vi "mainMultiColorWorm_2.vi"() -> ()   [LabVIEW 2017]
uses:
  globalUtilities.vi
  getComputerName.vi
  globalDevices.vi
panel:
  in  "piezo":bool
  in  "etl0_0 (piezo_0)":dbl
  out "curr exp time":dbl
  in  "abort":bool
  out "current image 3":u16[][](graph)
  out "current image 2":u16[][](graph)
  out "current image 1":u16[][](graph)
  out "current image 0":u16[][](graph)
  out "current channel":string
  out "current plane":i32
  in  "Strain name":string
  out "folder name":string
  in  "number of Z planes":i32=25
  in  "height of volume (um)":dbl=30.0
  in  "molecules":T1(array[cluster])=[{"molecule"="BFP", "exposureTimeMultiplier"=1.0}, {"molecule"="CyOFP", "exposureTimeMultiplier"=6.0}, {"molecule"="mCherry", "exposureTimeMultiplier"=4.0}, {"molecule"="mNeptune", "exposureTimeMultiplier"=5.0}]
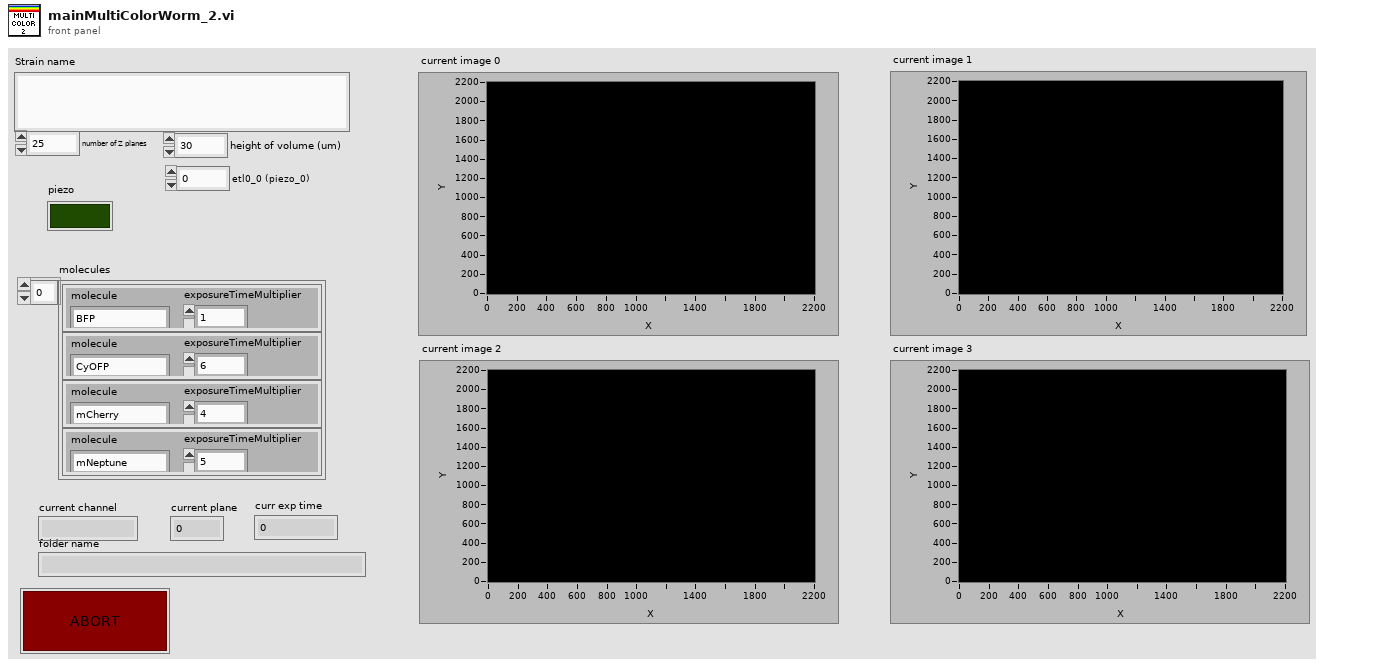
[diagram p1: front panel]
types:
  T1 = cluster{"molecule":string, "exposureTimeMultiplier":dbl}[]
  T2 = cluster{"height":i32, "width":i32, "datatype":i32}
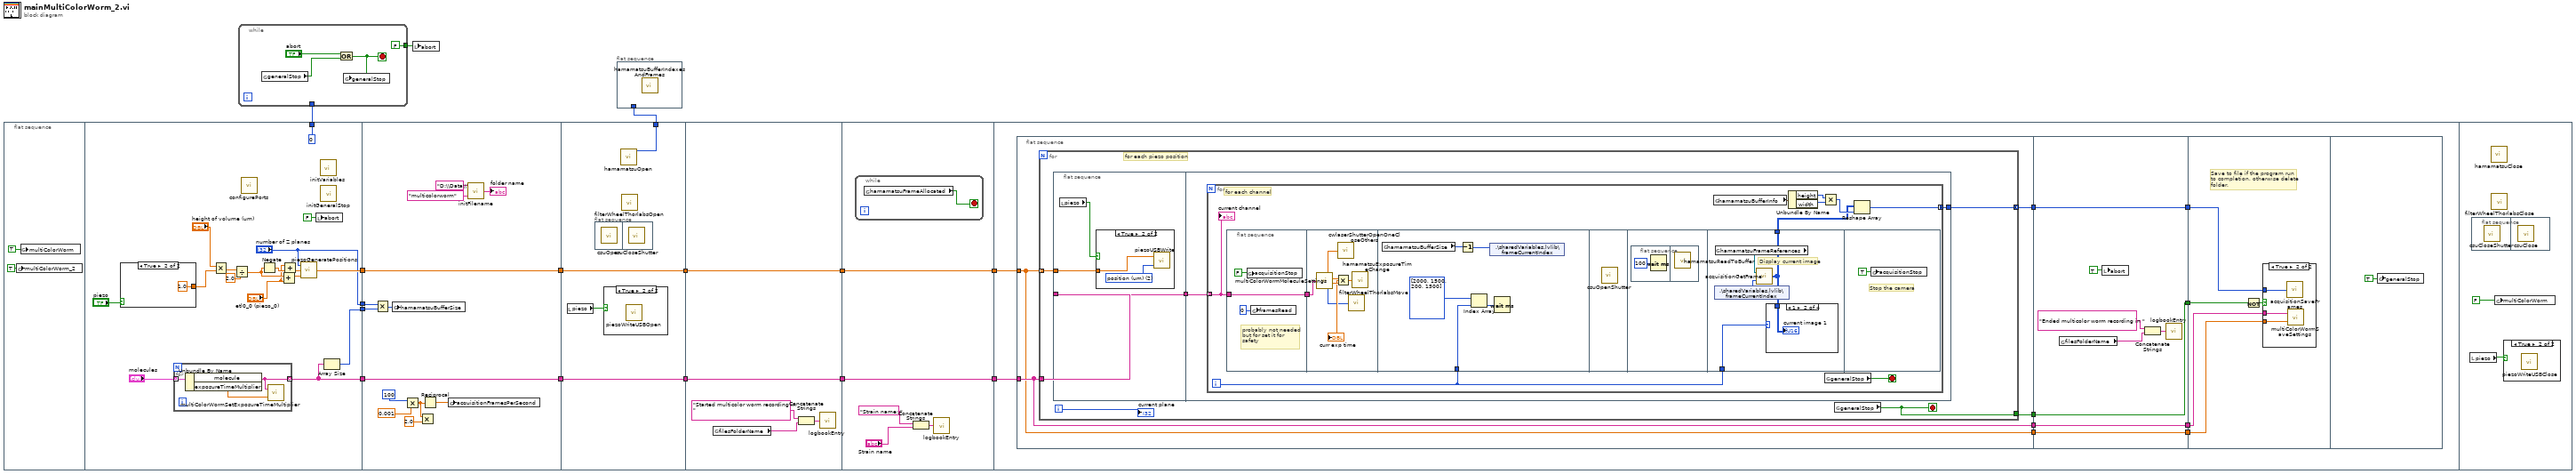
[diagram p0: block diagram]
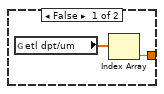
[diagram p2: hidden frame]
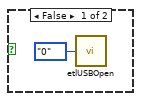
[diagram p3: hidden frame]
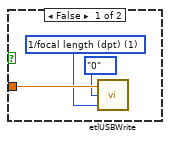
[diagram p4: hidden frame]
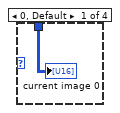
[diagram p5: hidden frame]
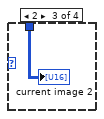
[diagram p6: hidden frame]
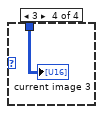
[diagram p7: hidden frame]
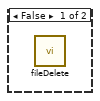
[diagram p8: hidden frame]
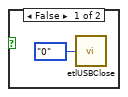
[diagram p9: hidden frame]
diagram:
  n1 = flat-sequence {
    tunnel: [w26] -> w15
    tunnel: [w34] -> w14
    tunnel: ["number of Z planes"] -> w13
    tunnel: [w33] -> w12
    tunnel: [0] -> w2
    tunnel: [w51] -> w11
    tunnel: w15 -> [w51]
    tunnel: [w50] -> w10
    tunnel: w14 -> [w50]
    tunnel: w13 -> [w48]
    tunnel: w12 -> [w47]
    tunnel: [w55] -> w9
    tunnel: [w56] -> w8
    tunnel: [w57] -> w3
    tunnel: w11 -> [w56]
    tunnel: w10 -> [w55]
    tunnel: w9 -> [w63]
    tunnel: [w63] -> w7
    tunnel: w8 -> [w62]
    tunnel: [w62] -> w6
    tunnel: w7 -> [w68]
    tunnel: [w68] -> w5
    tunnel: w6 -> [w67]
    tunnel: [w67] -> w4
    tunnel: w5 -> [w79]
    tunnel: w4 -> [w78]
    frame #0 {
      n2 = global write "globalUtilities.vi" "multiColorWorm_2"(TRUE ("multiColorWorm")) -> ()
      n3 = global write "globalUtilities.vi" "multiColorWorm"(TRUE ("multiColorWorm")) -> ()
    }
    frame #1 {
      n4 = case shown="True" "piezo" {
        tunnel: [w35 1.0 ("etl2UmPerV")] -> w25
        frame False {
          n5 = global read "globalDevices.vi" "etl dpt/um"() -> (w36:dbl[])
          n6 = Index Array(array=w36) -> (element=w35:dbl)  [unwired: 1 in]
        }
        frame True {
        }
      }
      n7 = for {
        tunnel: "molecules" -> [w40] mode=indexing
        tunnel: [w39] -> w26 mode=indexing
        n8 = Unbundle By Name(w40) -> ("molecule"=w39:string, "exposureTimeMultiplier"=w38:dbl)
        n9 = call "multiColorWormSetExposureTimeMultiplier.vi"("exposureTimeMultiplier"=w38, "molecule"=w39) -> ()  [unwired: 1 in]
      }
      n10 = Multiply(x="height of volume (um)", y=w25) -> (x*y=w29:dbl)
      n11 = Divide(x=w29, y=2.0) -> (x/y=w22:dbl)
      n12 = call "configurePorts.vi"() -> ()  [unwired: 12 in]
      n13 = Negate(x=w22) -> (-x=w23:dbl)
      n14 = Add(x=w22, y="etl0_0 (piezo_0)") -> (x+y=w20:dbl)
      n15 = Add(x="etl0_0 (piezo_0)", y=w23) -> (x+y=w21:dbl)
      n16 = call "piezoGeneratePositions.vi"("zf"=w20, "z0"=w21, "M"="number of Z planes") -> ("positions (z)"=w34:dbl[])
      n17 = local write "abort"(FALSE ("abort")) -> ()
      n18 = call "initVariables.vi"() -> ()  [unwired: 12 in]
      n19 = call "initGeneralStop.vi"() -> ()  [unwired: 1 in]
      n20 = Array Size(array=w26) -> (size(s)=w33:i32)
    }
    frame #2 {
      n21 = Multiply(x=w48, y=w47) -> (x*y=w49:i32)
      n22 = global write "globalDevices.vi" "hamamatsuBufferSize"(w49) -> ()
      n23 = Multiply(x=u16 100 ("exposure (ms)"), y=0.001) -> (x*y=w43:dbl)
      n24 = Multiply(x=w43, y=2.0) -> ()  [unwired: 1 out]
      n25 = Reciprocal(x=w43) -> (1/x=w52:dbl)
      n26 = global write "globalUtilities.vi" "acquisitionFramesPerSecond"(w52) -> ()
      n27 = call "initFilename.vi"("Experiment type"="multicolorworm", "Base disk and folder"="D:\\Data\\") -> ("folder name"=→"folder name":string)
    }
    frame #3 {
      n28 = local read "piezo"() -> (w54:bool)
      n29 = flat-sequence {
        frame #0 {
          n30 = call "csuOpen.vi"() -> ()  [unwired: 14 in, 2 out]
        }
        frame #1 {
          n31 = call "csuCloseShutter.vi"() -> ()  [unwired: 16 in]
        }
      }
      n32 = case shown="True" w54 {
        frame False {
          n33 = call "etlUSBOpen.vi"("lens"=enum16{"0", "1"}."0") -> ()  [unwired: 1 in, 1 out]
        }
        frame True {
          n34 = call "piezoWriteUSBOpen.vi"() -> ()  [unwired: 12 in]
        }
      }
      n35 = call "hamamatsuOpen.vi"() -> ("Handle out"=w57:u32)  [unwired: 3 out]
      n36 = call "filterWheelThorlabsOpen.vi"() -> ()  [unwired: 12 in]
    }
    frame #4 {
      n37 = global read "globalUtilities.vi" "filesFolderName"() -> (w60:string)
      n38 = Concatenate Strings("Started multicolor worm recording in ", w60) -> (w61:string)
      n39 = call "logbookEntry.vi"("Log book entry"=w61) -> ()  [unwired: 2 out]
    }
    frame #5 {
      n40 = while {
        stop <- w69 stop-if-true
        n41 = global read "globalDevices.vi" "hamamatsuFrameAllocated"() -> (w69:bool)
      }
      n42 = Concatenate Strings("Strain name: " ("string"), "Strain name") -> (w66:string)
      n43 = call "logbookEntry.vi"("Log book entry"=w66) -> ()  [unwired: 2 out]
    }
    frame #6 {
      n44 = flat-sequence {
        tunnel: w79 -> [w81]
        tunnel: w78 -> [w82]
        tunnel: [w83] -> w77
        tunnel: [w82] -> w75
        tunnel: [w81] -> w73
        tunnel: [w80] -> w71
        tunnel: w77 -> [w141]
        tunnel: [w141] -> w76
        tunnel: w75 -> [w140]
        tunnel: [w140] -> w74
        tunnel: w73 -> [w139]
        tunnel: [w139] -> w72
        tunnel: w71 -> [w134]
        tunnel: [w134] -> w70
        tunnel: w76 -> [w146]
        tunnel: w74 -> [w145]
        tunnel: w72 -> [w144]
        tunnel: w70 -> [w142]
        frame #0 {
          n45 = for {
            tunnel: w81 -> [w89] mode=indexing
            tunnel: w82 -> [w88]
            tunnel: [w87] -> w83 mode=concatenating
            tunnel: [w85] -> w80
            i -> [w86]
            stop <- w85 stop-if-true
            # "for each piezo position"
            n46 = flat-sequence {
              tunnel: w89 -> [w91]
              tunnel: w88 -> [w92]
              tunnel: [w92] -> w84
              tunnel: w84 -> [w99]
              tunnel: [w98] -> w87
              frame #0 {
                n47 = local read "piezo"() -> (w90:bool)
                n48 = case shown="True" w90 {
                  tunnel: w91 -> [w95 w96]
                  frame False {
                    w93 = u16 1 items=["position (um)", "1/focal length (dpt)"] ("mode")
                    n49 = call "etlUSBWrite.vi"("mode"=w93, "lens"=enum16{"0", "1"}."0", "input"=w95) -> ()  [unwired: 1 in]
                  }
                  frame True {
                    w97 = u16 2 items=["fractional", "voltage (V)", "position (um)"] ("mode")
                    n50 = call "piezoUSBWrite.vi"("mode"=w97, "position"=w96) -> ()  [unwired: 1 in]
                  }
                }
              }
              frame #1 {
                n51 = for {
                  tunnel: w99 -> [w101] mode=indexing
                  tunnel: [w103] -> w98 mode=concatenating
                  i -> [w100]
                  stop <- w102 stop-if-true
                  # "for each channel"
                  n52 = flat-sequence {
                    tunnel: w101 -> [w112]
                    tunnel: [w112] -> w109
                    tunnel: w109 -> [w118]
                    tunnel: w100 -> [w120]
                    tunnel: [w126] -> w104
                    tunnel: w100 -> [w127]
                    frame #0 {
                      # "probably not needed\nbut for set it for \nsafety"
                      n53 = global write "globalUtilities.vi" "acquisitionStop"(FALSE ("acquisitionStop")) -> ()
                      n54 = global write "globalUtilities.vi" "framesRead"(u32 0 ("framesRead")) -> ()
                    }
                    frame #1 {
                      n55 = call "multiColorWormMoleculeSettings.vi"("molecule"=w118) -> ("laserWavelength"=w114:dbl, "filter wheel position"=w113:u8, "exposure time (s)"=w116:dbl, "exposureTimeMultiplier"=w117:dbl)  [unwired: 2 out]
                      n56 = Multiply(x=w116, y=w117) -> (x*y=w115:dbl)
                      "curr exp time" <- w115
                      n57 = call "cwlaserShutterOpenOneCloseOthers.vi"("wavelength"=w114) -> ()  [unwired: 1 in]
                      n58 = call "filterWheelThorlabsMove.vi"("position"=w113) -> ()  [unwired: 1 in]
                      n59 = call "hamamatsuExposureTimeChange.vi"("Exposure time (s)"=w115) -> ()  [unwired: 1 out]
                    }
                    frame #2 {
                      n60 = global read "globalDevices.vi" "hamamatsuBufferSize"() -> (w123:i32)
                      n61 = Decrement(x=w123) -> (x-1=w122:i32)
                      n62 = Index Array(array=u32[] [2000, 1500, 200, 1500], index=w120) -> (element=w119:u32)
                      n63 = shared-variable ".\\sharedVariables.lvlib\\frameCurrentIndex"(w122) -> ()  [unwired: 1 in, 1 out]
                      n64 = Wait (ms)(milliseconds to wait=w119) -> ()  [unwired: 1 out]
                    }
                    frame #3 {
                      n65 = call "csuOpenShutter.vi"() -> ()  [unwired: 16 in]
                    }
                    frame #4 {
                      n66 = flat-sequence {
                        frame #0 {
                          n67 = Wait (ms)(milliseconds to wait=u32 100) -> ()  [unwired: 1 out]
                        }
                        frame #1 {
                          n68 = call "hamamatsuReadToBuffer.vi"() -> ()  [unwired: 12 in]
                        }
                      }
                    }
                    frame #5 {
                      # "Display current image"
                      n69 = shared-variable ".\\sharedVariables.lvlib\\frameCurrentIndex"() -> (w125:i32)  [unwired: 1 in, 1 out]
                      n70 = global read "globalDevices.vi" "hamamatsuFrameReferences"() -> (w128:refnum<data-value>[])
                      n71 = call "acquisitionGetFrame.vi"("index"=w125, "hamamatsuFrameReferences"=w128) -> ("frameOut"=w126:u16[][])
                      n72 = case shown="1" w127 {
                        tunnel: w126 -> [w129 w130 w131 w132]
                        frame 0, Default {
                          "current image 0" <- w129
                        }
                        frame 1 {
                          "current image 1" <- w130
                        }
                        frame 2 {
                          "current image 2" <- w131
                        }
                        frame 3 {
                          "current image 3" <- w132
                        }
                      }
                    }
                    frame #6 {
                      # "Stop the camera"
                      n73 = global write "globalUtilities.vi" "acquisitionStop"(TRUE ("acquisitionStop")) -> ()
                    }
                  }
                  n74 = global read "globalDevices.vi" "hamamatsuBufferInfo"() -> (w108:T2)
                  n75 = Unbundle By Name(w108) -> ("height"=w107:i32, "width"=w106:i32)
                  n76 = Multiply(x=w107, y=w106) -> (x*y=w105:i32)
                  n77 = global read "globalUtilities.vi" "generalStop"() -> (w102:bool)
                  n78 = Reshape Array(w104, w105) -> (w103:u16[])
                  "current channel" <- w101
                }
              }
            }
            n79 = global read "globalUtilities.vi" "generalStop"() -> (w85:bool)
            "current plane" <- w86
          }
        }
        frame #1 {
          n80 = global read "globalUtilities.vi" "filesFolderName"() -> (w138:string)
          n81 = local write "abort"(TRUE ("abort")) -> ()
          n82 = Concatenate Strings("Ended multicolor worm recording in ", w138) -> (w137:string)
          n83 = call "logbookEntry.vi"("Log book entry"=w137) -> ()  [unwired: 2 out]
        }
        frame #2 {
          # "Save to file if the program run\nto completion, otherwise delete\nfolder."
          n84 = Not(x=w142) -> (.not. x?=w143:bool)
          n85 = case shown="True" w143 {
            tunnel: w146 -> [_ w149]
            tunnel: w145 -> [_ w148]
            tunnel: w144 -> [_ w147]
            frame False {
              n86 = call "fileDelete.vi"() -> ()  [unwired: 12 in]
            }
            frame True {
              n87 = call "acquisitionSaveFrames.vi"("frames (1D)"=w149) -> ()  [unwired: 1 in]
              n88 = call "multiColorWormSaveSettings.vi"("piezoPosition"=w147, "moleculesSequence"=w148) -> ()  [unwired: 1 in]
            }
          }
        }
        frame #3 {
          n89 = global write "globalUtilities.vi" "generalStop"(TRUE ("generalStop")) -> ()
        }
      }
    }
    frame #7 {
      n90 = local read "piezo"() -> (w151:bool)
      n91 = flat-sequence {
        frame #0 {
          n92 = call "csuCloseShutter.vi"() -> ()  [unwired: 16 in]
        }
        frame #1 {
          n93 = call "csuClose.vi"() -> ()  [unwired: 12 in]
        }
      }
      n94 = call "hamamatsuClose.vi"() -> ()  [unwired: 1 out]
      n95 = call "filterWheelThorlabsClose.vi"() -> ()  [unwired: 12 in]
      n96 = global write "globalUtilities.vi" "multiColorWorm"(FALSE ("multiColorWorm")) -> ()
      n97 = case shown="True" w151 {
        frame False {
          n98 = call "etlUSBClose.vi"("lens"=enum16{"0", "1"}."0") -> ()  [unwired: 1 in]
        }
        frame True {
          n99 = call "piezoWriteUSBClose.vi"() -> ()  [unwired: 12 in]
        }
      }
    }
  }
  n100 = while {
    tunnel: w2 -> [_]
    tunnel: [FALSE] -> w1
    stop <- w156 stop-if-true
    n101 = global read "globalUtilities.vi" "generalStop"() -> (w155:bool)
    n102 = Or(x="abort", y=w155) -> (x .or. y?=w156:bool)
    n103 = global write "globalUtilities.vi" "generalStop"(w156) -> ()
  }
  n104 = local write "abort"(w1) -> ()
  n105 = flat-sequence {
    tunnel: w3 -> [_]
    frame #0 {
      n106 = call "hamamatsuBufferIndexesAndFrames.vi"() -> ()  [unwired: 12 in]
    }
  }
